vi "Rohde & Schwarz VNA Set Measurement.vi"(6 "Channel":i8=1 min=1 max=99 step=1, 7 "Rohde & Schwarz VNA":T1, 8 "error in (no error)":errorcluster, 9 "Conversion (Off)":T2, 10 "Measurement (S11)":T3, 11 "VISA Resource Name":refnum<visa-resource-name>) -> (0 "error out":errorcluster, 3 "dup VISA Resource Name":refnum<visa-resource-name>)   [LabVIEW 2011]
doc: "This VI for the HP8753B Network Analyzer sets the measurement."
uses:
  TypeDefs/Rohde & Schwarz VNA Measurement.ctl
  TypeDefs/Rohde & Schwarz VNA Conversion.ctl
  TypeDefs/Rohde & Schwarz VNA Instrument Info.ctl
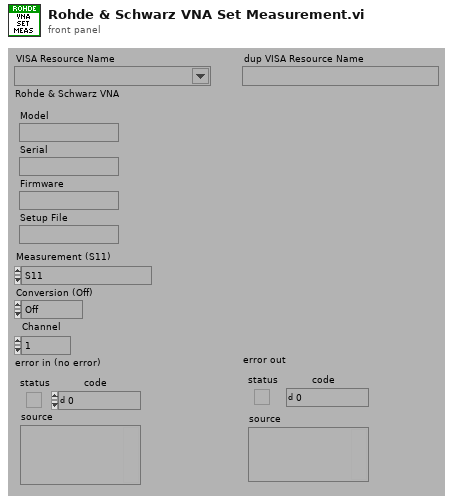
[diagram p1: front panel]
types:
  T1 = typedef "Rohde & Schwarz VNA Instrument Info.ctl" = cluster{"Model":string, "Serial":string, "Firmware":string, "Setup File":string}
  T2 = typedef "Rohde & Schwarz VNA Conversion.ctl" = enum16{"Off", "Fundamental", "Harmonic", "2nd Harmonic", "3rd Harmonic", "Mixer"}
  T3 = typedef "Rohde & Schwarz VNA Measurement.ctl" = enum32{"S11", "S12", "S21", "S22", "A1 Port 1 Source", "A1 Port 2 Source", "A2 Port 1 Source", "A2 Port 2 Source", "B1 Port 1 Source", "B1 Port 2 Source", "B2 Port 1 Source", "B2 Port 2 Source", "A1/A2 Port 1 Source", "A1/A2 Port 2 Source", "A1/B1 Port 1 Source", "A1/B1 Port 2 Source", "A1/B2 Port 1 Source", "A1/B2 Port 2 Source", "A2/A1 Port 1 Source", "A2/A1 Port 2 Source", "A2/B1 Port 1 Source", "A2/B1 Port 2 Source", "A2/B2 Port 1 Source", "A2/B2 Port 2 Source", "B1/A1 Port 1 Source", "B1/A1 Port 2 Source", "B1/A2 Port 1 Source", "B1/A2 Port 2 Source", "B1/B2 Port 1 Source", "B1/B2 Port 2 Source", "B2/A1 Port 1 Source", "B2/A1 Port 2 Source", "B2/A2 Port 1 Source", "B2/A2 Port 2 Source", "B2/B1 Port 1 Source", "B2/B1 Port 2 Source", "Z<-S11", "Z<-S12", "Z<-S21", "Z<-S22", "Y<-S11", "Y<-S12", "Y<-S21", "Y<-S22", "Z11", "Z12", "Z21", "Z22", "Y11", "Y12", "Y21", "Y22", "DC±1V", "DC±10V", "Unsupported"}
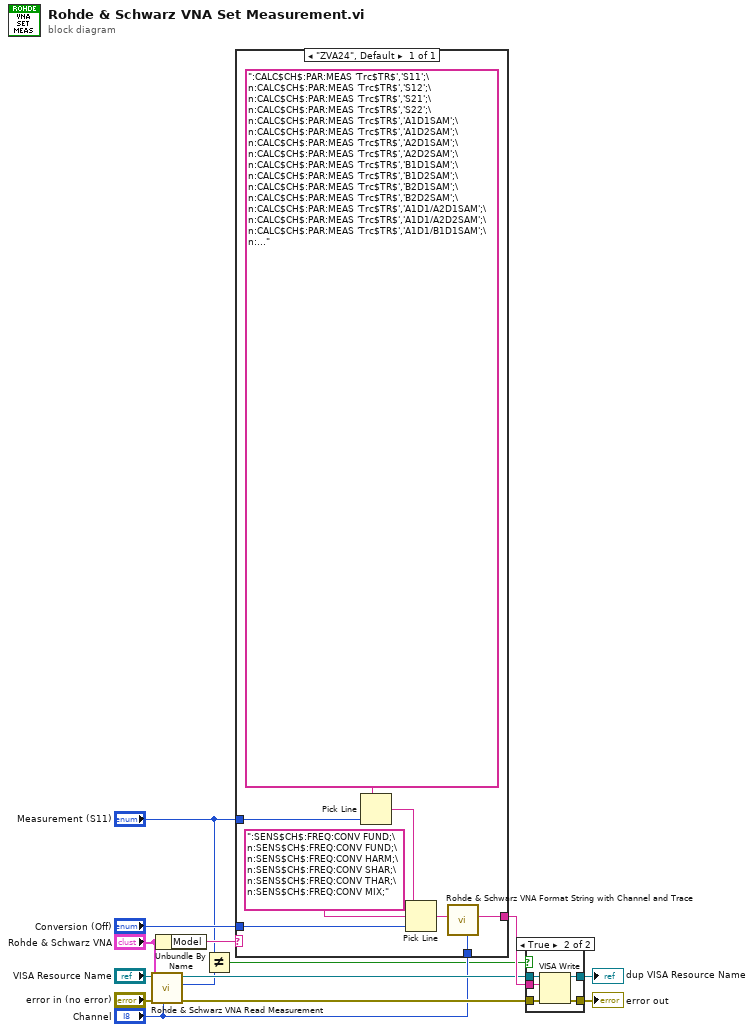
[diagram p0: block diagram]
diagram:
  n1 = call "Rohde & Schwarz VNA Read Measurement.vi"("Channel"="Channel", "Rohde & Schwarz VNA"="Rohde & Schwarz VNA", "error in (no error)"="error in (no error)", "VISA Resource Name"="VISA Resource Name") -> ("error out"=w7:errorcluster, "Measurement (S11)"=w6:T3, "dup VISA Resource Name"=w8:refnum<visa-resource-name>)  [unwired: 5 out]
  n2 = Unbundle By Name("Rohde & Schwarz VNA") -> ("Model"=w2:string)
  n3 = Not Equal?(x="Measurement (S11)", y=w6) -> (x != y?=w4:bool)
  n4 = case shown="\"ZVA24\", Default" w2 {
    tunnel: "Conversion (Off)" -> [w22]
    tunnel: [w17] -> w13
    tunnel: "Measurement (S11)" -> [w19]
    tunnel: "Channel" -> [w15]
    frame "ZVA24", Default {
      n5 = Pick Line(multi-line string=":CALC$CH$:PAR:MEAS 'Trc$TR$','S11';\n:CALC$CH$:PAR:MEAS 'Trc$TR$','S12';\n:CALC$CH$:PAR:MEAS 'Trc$TR$','S21';\n:CALC$CH$:PAR:MEAS 'Trc$TR$','S22';\n:CALC$CH$:PAR:MEAS 'Trc$TR$','A1D1SAM';\n:CALC$CH$:PAR:MEAS 'Trc$TR$','A1D2SAM';\n:CALC$CH$:PAR:MEAS 'Trc$TR$','A2D1SAM';\n:CALC$CH$:PAR:MEAS 'Trc$TR$','A2D2SAM';\n:CALC$CH$:PAR:MEAS 'Trc$TR$','B1D1SAM';\n:CALC$CH$:PAR:MEAS 'Trc$TR$','B1D2SAM';\n:CALC$CH$:PAR:MEAS 'Trc$TR$','B2D1SAM';\n:CALC$CH$:PAR:MEAS 'Trc$TR$','B2D2SAM';\n:CALC$CH$:PAR:MEAS 'Trc$TR$','A1D1/A2D1SAM';\n:CALC$CH$:PAR:MEAS 'Trc$TR$','A1D1/A2D2SAM';\n:CALC$CH$:PAR:MEAS 'Trc$TR$','A1D1/B1D1SAM';\n:CALC$CH$:PAR:MEAS 'Trc$TR$','A1D1/B1D2SAM';\n:CALC$CH$:PAR:MEAS 'Trc$TR$','A1D1/B2D1SAM';\n:CALC$CH$:PAR:MEAS 'Trc$TR$','A1D1/B2D2SAM';\n:CALC$CH$:PAR:MEAS 'Trc$TR$','A2D1/A1D1SAM';\n:CALC$CH$:PAR:MEAS 'Trc$TR$','A2D1/A1D2SAM';\n:CALC$CH$:PAR:MEAS 'Trc$TR$','A2D1/B1D1SAM';\n:CALC$CH$:PAR:MEAS 'Trc$TR$','A2D1/B1D2SAM';\n:CALC$CH$:PAR:MEAS 'Trc$TR$','A2D1/B2D1SAM';\n:CALC$CH$:PAR:MEAS 'Trc$TR$','A2D1/B2D2SAM';\n:CALC$CH$:PAR:MEAS 'Trc$TR$','B1D1/A1D1SAM';\n:CALC$CH$:PAR:MEAS 'Trc$TR$','B1D1/A1D2SAM';\n:CALC$CH$:PAR:MEAS 'Trc$TR$','B1D1/A2D1SAM';\n:CALC$CH$:PAR:MEAS 'Trc$TR$','B1D1/A2D2SAM';\n:CALC$CH$:PAR:MEAS 'Trc$TR$','B1D1/B2D1SAM';\n:CALC$CH$:PAR:MEAS 'Trc$TR$','B1D1/B2D2SAM';\n:CALC$CH$:PAR:MEAS 'Trc$TR$','B2D1/A1D1SAM';\n:CALC$CH$:PAR:MEAS 'Trc$TR$','B2D1/A1D2SAM';\n:CALC$CH$:PAR:MEAS 'Trc$TR$','B2D1/A2D1SAM';\n:CALC$CH$:PAR:MEAS 'Trc$TR$','B2D1/A2D2SAM';\n:CALC$CH$:PAR:MEAS 'Trc$TR$','B2D1/B1D1SAM';\n:CALC$CH$:PAR:MEAS 'Trc$TR$','B2D1/B1D2SAM';\n:CALC$CH$:PAR:MEAS 'Trc$TR$','Z-S11';\n:CALC$CH$:PAR:MEAS 'Trc$TR$','Z-S12';\n:CALC$CH$:PAR:MEAS 'Trc$TR$','Z-S21';\n:CALC$CH$:PAR:MEAS 'Trc$TR$','Z-S22';\n:CALC$CH$:PAR:MEAS 'Trc$TR$','Y-S11';\n:CALC$CH$:PAR:MEAS 'Trc$TR$','Y-S12';\n:CALC$CH$:PAR:MEAS 'Trc$TR$','Y-S21';\n:CALC$CH$:PAR:MEAS 'Trc$TR$','Y-S22';\n:CALC$CH$:PAR:MEAS 'Trc$TR$','Z11';\n:CALC$CH$:PAR:MEAS 'Trc$TR$','Z12';\n:CALC$CH$:PAR:MEAS 'Trc$TR$','Z21';\n:CALC$CH$:PAR:MEAS 'Trc$TR$','Z22';\n:CALC$CH$:PAR:MEAS 'Trc$TR$','Y11';\n:CALC$CH$:PAR:MEAS 'Trc$TR$','Y12';\n:CALC$CH$:PAR:MEAS 'Trc$TR$','Y21';\n:CALC$CH$:PAR:MEAS 'Trc$TR$','Y22';\n:CALC$CH$:PAR:MEAS 'Trc$TR$','DC±1V';\n:CALC$CH$:PAR:MEAS 'Trc$TR$','DC±10V';\nUNSUPPORTED", line index=w19) -> (output string=w16:string)  [unwired: 1 out]
      n6 = Pick Line(string ("")=w16, multi-line string=":SENS$CH$:FREQ:CONV FUND;\n:SENS$CH$:FREQ:CONV FUND;\n:SENS$CH$:FREQ:CONV HARM;\n:SENS$CH$:FREQ:CONV SHAR;\n:SENS$CH$:FREQ:CONV THAR;\n:SENS$CH$:FREQ:CONV MIX;", line index=w22) -> (output string=w18:string)
      n7 = call "Rohde & Schwarz VNA Format String with Channel and Trace.vi"("Trace"=w15, "String"=w18) -> ("String Out"=w17:string)  [unwired: 1 in, 6 out]
    }
  }
  n8 = case shown="True" w4 {
    tunnel: w13 -> [_ w29]
    tunnel: [w23 w28] -> w12
    tunnel: [w24 w27] -> w11
    tunnel: w8 -> [w23 w26]
    tunnel: w7 -> [w24 w25]
    frame False {
    }
    frame True {
      n9 = VISA Write(VISA resource name=w26, write buffer=w29, error in (no error)=w25) -> (VISA resource name out=w28:refnum<visa-resource-name>, error out=w27:errorcluster)  [unwired: 1 out]
    }
  }
  "dup VISA Resource Name" <- w12
  "error out" <- w11
